vi "Periodic Tasks.vi"(8 "error in":errorcluster) -> ()   [LabVIEW 2023]
doc: "This VI runs in parallel to other tasks. It can contain as many user-defined periodic loops as you need. These can carry out PID or other sorts of timed response."
uses:
  <vilib>/Rock Robotics/WPI/Utilities/WPI_GetSetVariantRefNum.vi
  <vilib>/Rock Robotics/Network Tables/NT Write Integer Array.vi
  <vilib>/Rock Robotics/Network Tables/NT Write Float.vi
panel:
  out "Pitch":dbl
  out "Roll":dbl
  out "Yaw":dbl
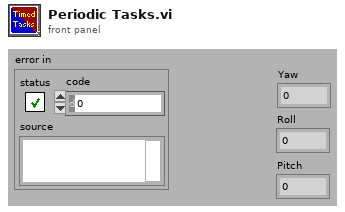
[diagram p1: front panel]
types:
  T1 = typedef "WPI_JoystickDevRef.ctl" = cluster{"Device":T2}
  T2 = typedef "WPI_JoystickDeviceEnum.ctl" = enum16{"USB 0", "USB 1", "USB 2", "USB 3", "USB 4", "USB 5"}
  T3 = typedef "WPI_RobotDriveDevRef.ctl" = cluster{"DevStatus":errorcluster, "Motors[]":T4[], "Square Inputs":bool, "Max Output":dbl}
  T4 = typedef "WPI_MotorControlDeviceRef.ctl" = cluster{"DeviceStatus":errorcluster, "Type":T5, "PWM":cluster{"PWM Channel":T6, "DeadBand":T7}, "CAN":cluster{"Device Number":u8, "SetOutput VI Ref":variant, "GetOutput VI Ref":variant, "Enable VI Ref":variant, "Disable VI Ref":variant, "Data":variant}, "Invert":bool, "DIO PWM":cluster{"PWM \"Enable\" Channel":T6, "DIOChannel":T8, "PWM Rate":dbl}}
  T5 = typedef "WPI_MotorControlType.ctl" = enum16{"PWM", "CAN", "DIO PWM"}
  T6 = typedef "FPGA_DIOPWMChannel.ctl" = enum8{"PWM 0", "PWM 1", "PWM 2", "PWM 3", "PWM 4", "PWM 5", "PWM 6", "PWM 7", "PWM 8", "PWM 9", "PWM MXP 0", "PWM MXP 1", "PWM MXP 2", "PWM MXP 3", "PWM MXP 4", "PWM MXP 5", "PWM MXP 6", "PWM MXP 7", "PWM MXP 8", "PWM MXP 9", "Invalid"}
  T7 = typedef "WPI_PWMDeadband.ctl" = cluster{"Name":string, "maxPositivePwm":i32, "minPositivePwm":i32, "centerPwm":i32, "maxNegativePwm":i32, "minNegativePwm":i32, "angularRange":u16}
  T8 = typedef "FPGA_DIOChannel.ctl" = enum8{"DIO 0", "DIO 1", "DIO 2", "DIO 3", "DIO 4", "DIO 5", "DIO 6", "DIO 7", "DIO 8", "DIO 9", "DIO MXP 0", "DIO MXP 1", "DIO MXP 2", "DIO MXP 3", "DIO MXP 4", "DIO MXP 5", "DIO MXP 6", "DIO MXP 7", "DIO MXP 8", "DIO MXP 9", "DIO MXP 10", "DIO MXP 11", "DIO MXP 12", "DIO MXP 13", "DIO MXP 14", "DIO MXP 15", "SPI Port CS1", "SPI Port CS2", "SPI Port CS3", "SPI Port MISO", "SPI Port MOSI", "Invalid"}
  T9 = cluster{"JoystickDevRef":T1, "RobotDriveDevRef":T3}
  T10 = cluster{"Yaw":dbl, "Roll":dbl, "Pitch":dbl, "Heading":dbl, "Fused Heading":dbl}
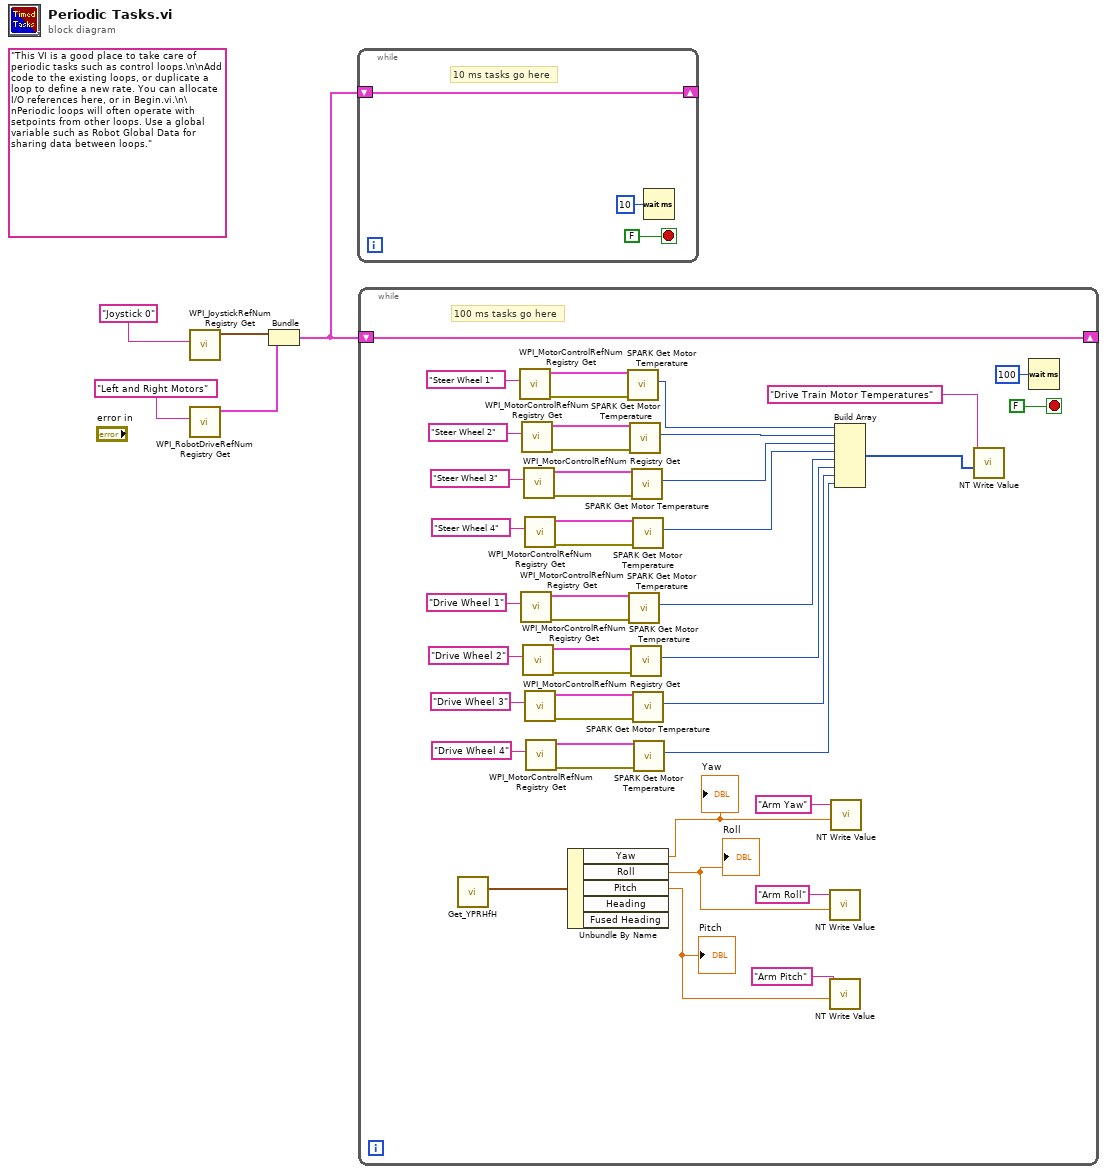
[diagram p0: block diagram]
diagram:
  (unwired) "This VI is a good place to take care of periodic tasks such as control loops.\n\nAdd code to the existing loops, or duplicate a loop to define a new rate. You can allocate I/O references here, or in Begin.vi.\n\nPeriodic loops will often operate with setpoints from other loops. Use a global variable such as Robot Global Data for sharing data between loops."
  n1 = call <vilib>:"WPI_JoystickRefNum Registry Get.vi"("refnum name"="Joystick 0") -> ("JoystickDevRef"=w3:T1)  [unwired: 1 in, 9 out]
  n2 = call <vilib>:"WPI_RobotDriveRefNum Registry Get.vi"("refnum name"="Left and Right Motors") -> ("RobotDriveDevRef"=w2:T3)  [unwired: 1 in, 9 out]
  n3 = Bundle("JoystickDevRef"=w3, "RobotDriveDevRef"=w2) -> (w1:T9)  [unwired: 1 out]
  n4 = while {
    shift-right: [w6] -> _
    shift-left: w1 -> [w6]
    stop <- FALSE stop-if-true
    # "10 ms tasks go here"
    n5 = Wait (ms)(milliseconds to wait=u32 10) -> ()  [unwired: 1 out]
  }
  n6 = while {
    shift-right: [w50] -> _
    shift-left: w1 -> [w50]
    stop <- FALSE stop-if-true
    # "100 ms tasks go here"
    n7 = call <vilib>:"Get_YPRHfH.vi"() -> ("YRPHfH"=w15:T10)  [unwired: 11 in]
    n8 = call <vilib>:"WPI_MotorControlRefNum Registry Get.vi"("refnum name"="Steer Wheel 1") -> ("error out"=w47:errorcluster, "MotorControlDevRef"=w48:T4)  [unwired: 9 in]
    n9 = call <vilib>:"WPI_MotorControlRefNum Registry Get.vi"("refnum name"="Drive Wheel 1") -> ("error out"=w35:errorcluster, "MotorControlDevRef"=w36:T4)  [unwired: 9 in]
    n10 = call <vilib>:"WPI_MotorControlRefNum Registry Get.vi"("refnum name"="Steer Wheel 2") -> ("error out"=w44:errorcluster, "MotorControlDevRef"=w45:T4)  [unwired: 9 in]
    n11 = call <vilib>:"WPI_MotorControlRefNum Registry Get.vi"("refnum name"="Drive Wheel 2") -> ("error out"=w32:errorcluster, "MotorControlDevRef"=w33:T4)  [unwired: 9 in]
    n12 = call <vilib>:"WPI_MotorControlRefNum Registry Get.vi"("refnum name"="Steer Wheel 3") -> ("error out"=w41:errorcluster, "MotorControlDevRef"=w42:T4)  [unwired: 9 in]
    n13 = call <vilib>:"WPI_MotorControlRefNum Registry Get.vi"("refnum name"="Steer Wheel 4") -> ("error out"=w38:errorcluster, "MotorControlDevRef"=w39:T4)  [unwired: 9 in]
    n14 = call <vilib>:"WPI_MotorControlRefNum Registry Get.vi"("refnum name"="Drive Wheel 3") -> ("error out"=w29:errorcluster, "MotorControlDevRef"=w30:T4)  [unwired: 9 in]
    n15 = call <vilib>:"WPI_MotorControlRefNum Registry Get.vi"("refnum name"="Drive Wheel 4") -> ("error out"=w26:errorcluster, "MotorControlDevRef"=w27:T4)  [unwired: 9 in]
    n16 = Unbundle By Name(w15) -> ("Yaw"=w11:dbl, "Roll"=w10:dbl, "Pitch"=w9:dbl)  [unwired: 2 out]
    "Yaw" <- w11
    "Roll" <- w10
    "Pitch" <- w9
    n17 = call <vilib>:"SPARK Get Motor Temperature.vi"("error in (no error)"=w47, "MotorControlDevRef in"=w48) -> ("Motor Temperature"=w25:u8)  [unwired: 6 in, 3 out]
    n18 = call <vilib>:"SPARK Get Motor Temperature.vi"("error in (no error)"=w35, "MotorControlDevRef in"=w36) -> ("Motor Temperature"=w21:u8)  [unwired: 6 in, 3 out]
    n19 = call <vilib>:"SPARK Get Motor Temperature.vi"("error in (no error)"=w44, "MotorControlDevRef in"=w45) -> ("Motor Temperature"=w24:u8)  [unwired: 6 in, 3 out]
    n20 = call <vilib>:"SPARK Get Motor Temperature.vi"("error in (no error)"=w32, "MotorControlDevRef in"=w33) -> ("Motor Temperature"=w20:u8)  [unwired: 6 in, 3 out]
    n21 = call <vilib>:"SPARK Get Motor Temperature.vi"("error in (no error)"=w41, "MotorControlDevRef in"=w42) -> ("Motor Temperature"=w23:u8)  [unwired: 6 in, 3 out]
    n22 = call <vilib>:"SPARK Get Motor Temperature.vi"("error in (no error)"=w38, "MotorControlDevRef in"=w39) -> ("Motor Temperature"=w22:u8)  [unwired: 6 in, 3 out]
    n23 = call <vilib>:"SPARK Get Motor Temperature.vi"("error in (no error)"=w29, "MotorControlDevRef in"=w30) -> ("Motor Temperature"=w19:u8)  [unwired: 6 in, 3 out]
    n24 = call <vilib>:"SPARK Get Motor Temperature.vi"("error in (no error)"=w26, "MotorControlDevRef in"=w27) -> ("Motor Temperature"=w18:u8)  [unwired: 6 in, 3 out]
    n25 = call-poly <vilib>:"NT Write Value.vi"("value"=w10, "name"="Arm Roll") -> ()  [unwired: 9 in, 1 out]
    n26 = call-poly <vilib>:"NT Write Value.vi"("value"=w9, "name"="Arm Pitch") -> ()  [unwired: 9 in, 1 out]
    n27 = call-poly <vilib>:"NT Write Value.vi"("value"=w11, "name"="Arm Yaw") -> ()  [unwired: 9 in, 1 out]
    n28 = Build Array(w25, w24, w23, w22, w21, w20, w19, w18) -> (w17:u8[])
    n29 = call-poly <vilib>:"NT Write Value.vi"("value"=w17, "name"="Drive Train Motor Temperatures") -> ()  [unwired: 9 in, 1 out]
    n30 = Wait (ms)(milliseconds to wait=u32 100) -> ()  [unwired: 1 out]
  }
